vi "niFPGA Decimation CU.vi"(7 "reset":bool, 11 "dataRDYIn":bool) -> (0 "idle?":bool, 1 "dataReady?":bool, 2 "read FIFO?":bool, 3 "write FIFO?":bool, 5 "coef idx":u16)   [LabVIEW 2017]
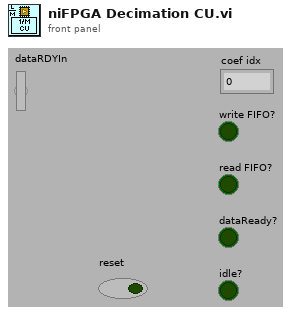
[diagram p1: front panel]
types:
  T1 = cluster{"kChanCnt":fxp<+,1,1>, "kPhaseCnt":fxp<+,2,2>, "kMacCnt":fxp<+,5,5>, "kCoefIdx":fxp<+,7,7>, "idle?":bool, "dataReady?":bool, "first run?":bool, "read FIFO?":bool, "write FIFO?":bool}
  T2 = cluster{"kTotalChan-1":fxp<+,1,1>, "kTotalPhase-1":fxp<+,2,2>, "kTapsPerPhase-1":fxp<+,5,5>}
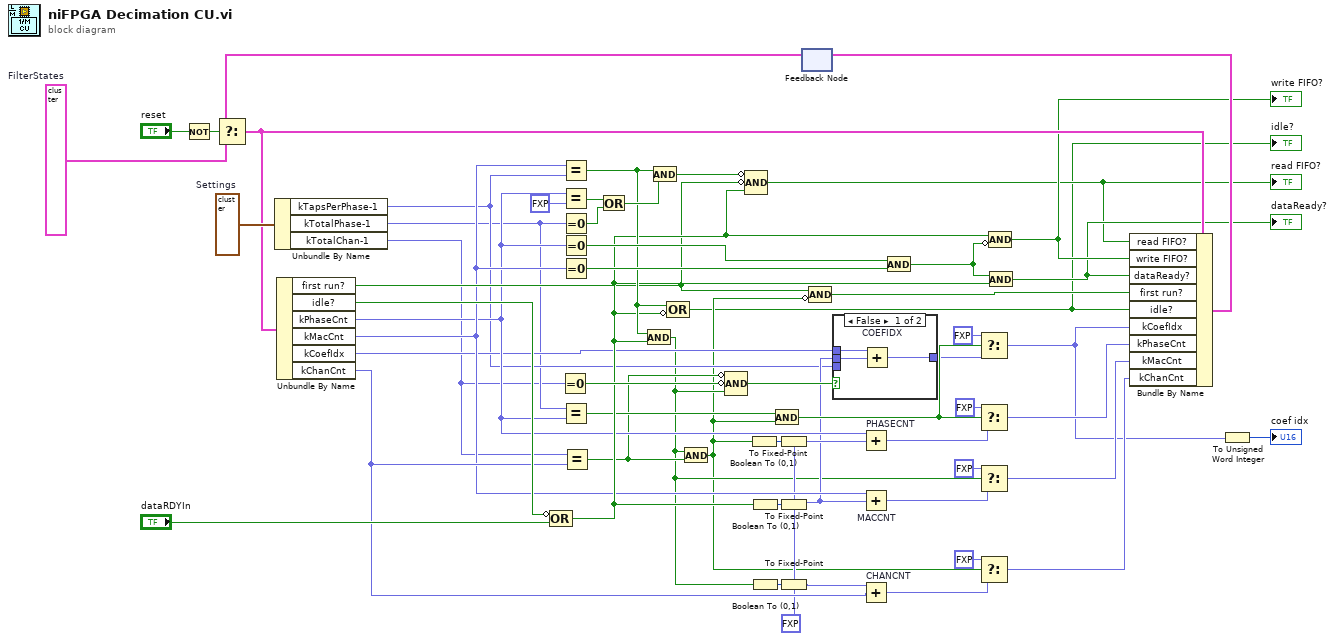
[diagram p0: block diagram]
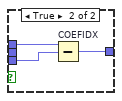
[diagram p2: hidden frame]
diagram:
  w6 = T1 {"kChanCnt"=0.0, "kPhaseCnt"=0.0, "kMacCnt"=0.0, "kCoefIdx"=0.0, "idle?"=TRUE, "dataReady?"=FALSE, "first run?"=TRUE, "read FIFO?"=FALSE, "write FIFO?"=FALSE}  # FilterStates
  w22 = fxp<+,1,1> 0.0 ("fixed-point type")
  w23 = T2 {"kTotalChan-1"=0.0, "kTotalPhase-1"=1.0, "kTapsPerPhase-1"=25.0}  # Settings
  n1 = Not(x="reset") -> (.not. x?=w12:bool)
  n2 = Unbundle By Name(w23) -> ("kTapsPerPhase-1"=w29:fxp<+,5,5>, "kTotalPhase-1"=w28:fxp<+,2,2>, "kTotalChan-1"=w27:fxp<+,1,1>)
  n3 = Equal To 0?(x=w27) -> (x = 0?=w46:bool)
  n4 = Equal To 0?(x=w28) -> (x = 0?=w52:bool)
  n5 = feedback #1() -> (w8:T1)  [unwired: 1 out]
  n6 = Select(t=w8, s=w12, f=w6) -> (s? t:f=w7:T1)
  n7 = Unbundle By Name(w7) -> ("first run?"=w42:bool, "idle?"=w43:bool, "kPhaseCnt"=w37:fxp<+,2,2>, "kMacCnt"=w38:fxp<+,5,5>, "kCoefIdx"=w34:fxp<+,7,7>, "kChanCnt"=w39:fxp<+,1,1>)
  n8 = Compound Arithmetic op=OR(invert w43, "dataRDYIn") -> (w45:bool)
  n9 = Equal?(x=w38, y=w29) -> (x = y?=w48:bool)
  n10 = Equal?(x=w37, y=fxp<+,1,1> 1.0) -> (x = y?=w53:bool)
  n11 = Equal To 0?(x=w37) -> (x = 0?=w55:bool)
  n12 = Equal To 0?(x=w38) -> (x = 0?=w54:bool)
  n13 = Equal?(x=w28, y=w37) -> (x = y?=w36:bool)
  n14 = Equal?(x=w27, y=w39) -> (x = y?=w32:bool)
  n15 = Or(x=w53, y=w52) -> (x .or. y?=w50:bool)
  n16 = And(x=w48, y=w45) -> (x .and. y?=w18:bool)
  n17 = And(x=w48, y=w50) -> (x .and. y?=w41:bool)
  n18 = Compound Arithmetic op=OR(w48, invert w45) -> (w2:bool)
  "idle?" <- w2
  n19 = And(x=w18, y=w32) -> (x .and. y?=w17:bool)
  n20 = Compound Arithmetic op=AND(invert w32, invert w46, w18) -> (w47:bool)
  n21 = Compound Arithmetic op=AND(invert w41, invert w42, w45) -> (w3:bool)
  "read FIFO?" <- w3
  n22 = Boolean To (0,1)(Boolean=w17) -> (0, 1=w56:i16)
  n23 = Boolean To (0,1)(Boolean=w45) -> (0, 1=w58:i16)
  n24 = Boolean To (0,1)(Boolean=w18) -> (0, 1=w31:i16)
  n25 = And(x=w36, y=w17) -> (x .and. y?=w35:bool)
  n26 = To Fixed-Point(fixed-point type=w22, number=w56) -> (fixed-point=w40:fxp<+,1,1>)
  n27 = To Fixed-Point(fixed-point type=w22, number=w58) -> (fixed-point=w33:fxp<+,1,1>)
  n28 = To Fixed-Point(fixed-point type=w22, number=w31) -> (fixed-point=w30:fxp<+,1,1>)
  n29 = Compound Arithmetic op=AND(w42, invert w17) -> (w51:bool)
  n30 = case shown="False" w47 {
    tunnel: w29 -> [_ w65]
    tunnel: [w60 w63] -> w11
    tunnel: w34 -> [w62 w64]
    tunnel: w33 -> [w61 _]
    frame False {
      n31 = Add "COEFIDX"(x=w62, y=w61) -> (x+y=w60:fxp<+,7,7>)
    }
    frame True {
      n32 = Subtract "COEFIDX"(x=w64, y=w65) -> (x-y=w63:fxp<+,7,7>)
    }
  }
  n33 = Add "PHASECNT"(x=w37, y=w40) -> (x+y=w15:fxp<+,2,2>)
  n34 = Add "MACCNT"(x=w38, y=w33) -> (x+y=w16:fxp<+,5,5>)
  n35 = Add "CHANCNT"(x=w30, y=w39) -> (x+y=w14:fxp<+,1,1>)
  n36 = And(x=w55, y=w54) -> (x .and. y?=w44:bool)
  n37 = Select(t=fxp<+,1,1> 0.0, s=w35, f=w11) -> (s? t:f=w1:fxp<+,7,7>)
  n38 = Select(t=fxp<+,1,1> 0.0, s=w35, f=w15) -> (s? t:f=w26:fxp<+,2,2>)
  n39 = Select(t=fxp<+,1,1> 0.0, s=w18, f=w16) -> (s? t:f=w25:fxp<+,5,5>)
  n40 = Select(t=fxp<+,1,1> 0.0, s=w17, f=w14) -> (s? t:f=w24:fxp<+,1,1>)
  n41 = And(x=w44, y=w45) -> (x .and. y?=w4:bool)
  "dataReady?" <- w4
  n42 = Compound Arithmetic op=AND(w45, invert w44) -> (w5:bool)
  "write FIFO?" <- w5
  n43 = Bundle By Name(cluster=w7, "read FIFO?"=w3, "write FIFO?"=w5, "dataReady?"=w4, "first run?"=w51, "idle?"=w2, "kCoefIdx"=w1, "kPhaseCnt"=w26, "kMacCnt"=w25, "kChanCnt"=w24) -> (w10:T1)
  n44 = feedback-in #1(w10) -> ()
  n45 = To Unsigned Word Integer(number=w1) -> (unsigned 16bit integer=→"coef idx":u16)
